vi "Open_Instr.vi"(8 "error in (no error)":errorcluster caption="entrée d'erreur (pas d'erreur)", 11 "Class Relay_Board en entrée":refnum<class "Class Instrument UART.lvclass">) -> (0 "error out":errorcluster caption="sortie d'erreur", 3 "Class Relay_Board en Sortie":refnum<class "Class Instrument UART.lvclass">)   [LabVIEW 2020, in "Library Instrument & Equipement.lvlib" / "Library Instruments.lvlib" / "Class Instrument UART.lvclass"]
uses:
  Class Instrument UART.lvclass
  Class Instrument UART.lvclass/Class Instrument UART.ctl
  Instrument (Default)/Class Instrument (Default).lvclass
  UART/UART (Default)/Class UART (Default).lvclass
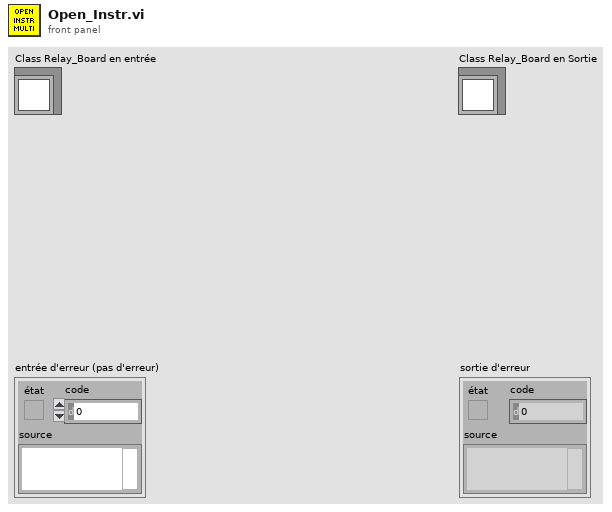
[diagram p1: front panel]
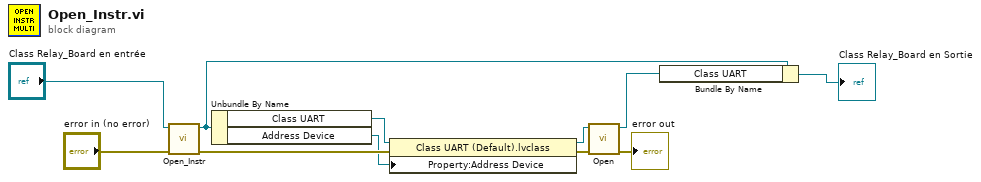
[diagram p0: block diagram]
diagram:
  n1 = call-parent "Open_Instr.vi"("error in (no error)"="error in (no error)", "Class Multimeter (Default) en entrée"="Class Relay_Board en entrée") -> ("error out"=w9:errorcluster, "Class Multimeter (Default) en sortie"=w7:refnum<class "Class Instrument UART.lvclass">)  [unwired: 8 in]
  n2 = Unbundle By Name(w7) -> ("Class UART"=w8:refnum<class "Class UART (Default).lvclass">, "Address Device"=w1:refnum<visa-resource-name>)
  n3 = property class="Class UART (Default).lvclass"(reference=w8, error in=w9, "Property:Address Device"=w1) -> (reference out=w3:refnum<class "Class UART (Default).lvclass">, error out=w5:errorcluster)
  n4 = call-dynamic "Open.vi"("error in (no error)"=w5, "Class UART (Default) en entrée"=w3) -> ("error out"=→"error out":errorcluster, "Class UART (Default) en sortie"=w2:refnum<class "Class UART (Default).lvclass">)  [unwired: 8 in]
  n5 = Bundle By Name(cluster=w7, "Class UART"=w2) -> (→"Class Relay_Board en Sortie":refnum<class "Class Instrument UART.lvclass">)
